vi "set_rotary_stage_voltage.vi"(6 "rotary voltage":dbl format="%0.2f", 7 "rotary voltage channel":tag, 10 "minimum value":dbl=-10.0 format="%0.2f", 11 "maximum value":dbl=10.0 format="%0.2f") -> ()   [LabVIEW 2019]
uses:
  <vilib>/DAQmx/write.llb/DAQmx Write (Analog DBL 1Chan 1Samp).vi
  <vilib>/DAQmx/create/channels.llb/DAQmx Create Channel (AO-Voltage-Basic).vi
  <vilib>/DAQmx/miscellaneous.llb/DAQmx Fill In Error Info.vi
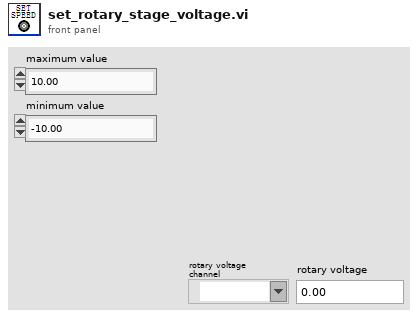
[diagram p1: front panel]
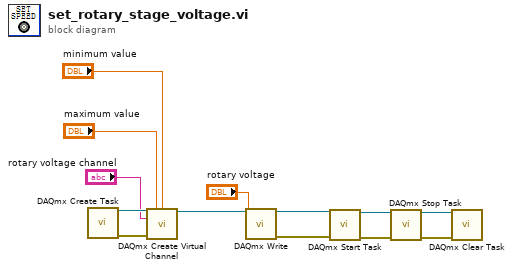
[diagram p0: block diagram]
diagram:
  n1 = call <vilib>:"DAQmx Create Task.vi"() -> ("task out"=w13:refnum<k21>, "error out"=w12:errorcluster)  [unwired: 14 in]
  n2 = call-poly <vilib>:"DAQmx Create Virtual Channel.vi"("task in"=w13, "maximum value"="maximum value", "minimum value"="minimum value", "physical channels"="rotary voltage channel", "error in"=w12) -> ("task out"=w11:refnum<k21>)  [unwired: 9 in, 1 out]
  n3 = call-poly <vilib>:"DAQmx Write.vi"("task/channels in"=w11, "data"="rotary voltage") -> ("task out"=w9:refnum<k21>, "error out"=w8:errorcluster)  [unwired: 11 in, 1 out]
  n4 = call <vilib>:"DAQmx Start Task.vi"("task/channels in"=w9, "error in"=w8) -> ("task out"=w7:refnum<k21>, "error out"=w6:errorcluster)  [unwired: 12 in]
  n5 = call <vilib>:"DAQmx Stop Task.vi"("task/channels in"=w7, "error in"=w6) -> ("task out"=w5:refnum<k21>, "error out"=w4:errorcluster)  [unwired: 12 in]
  n6 = call <vilib>:"DAQmx Clear Task.vi"("task in"=w5, "error in"=w4) -> ()  [unwired: 13 in, 1 out]
